vi "Read Data Titles.vi"(8 "error in (no error)":errorcluster, 11 "Device in":refnum<class "Cryo-Con-22C.lvclass">) -> (0 "error out":errorcluster, 2 "Data titles":string[](array[string])=["CRYO CHA"], 3 "Device out":refnum<class "Cryo-Con-22C.lvclass">)   [LabVIEW 2015, in "Cryo-Con-22C.lvclass"]
uses:
  Cryo-Con-22C.lvclass
  Cryo-Con Front Panel Data.ctl
  Cryo-con Heater Ranges.ctl
  Cry-Con Loop Type.ctl
  OO Devices/Device/Read Control Panel Loaded.vi
  OO Devices/Device/Read Controls Snapshot.vi
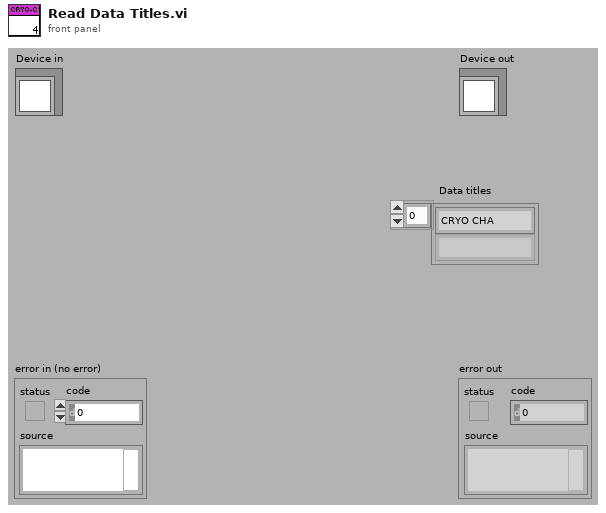
[diagram p1: front panel]
types:
  T1 = typedef "Cryo-Con Front Panel Data.ctl" = cluster{"Channels to measure":string[], "Record heater":bool, "Set point":dbl, "Heater Range":T2, "Control":bool, "Loop type":T3, "Ramp rate,\n K/min":dbl, "Control Channel":string, "P":dbl, "I":dbl, "D":dbl, "Manual %":u16}
  T2 = typedef "Cryo-con Heater Ranges.ctl" = enum16{"25W", "2.5W", "0.25W"}
  T3 = typedef "Cry-Con Loop Type.ctl" = enum16{"Off", "PID", "Manual", "PID Table", "PID Ramp", "PID Table Ramp"}
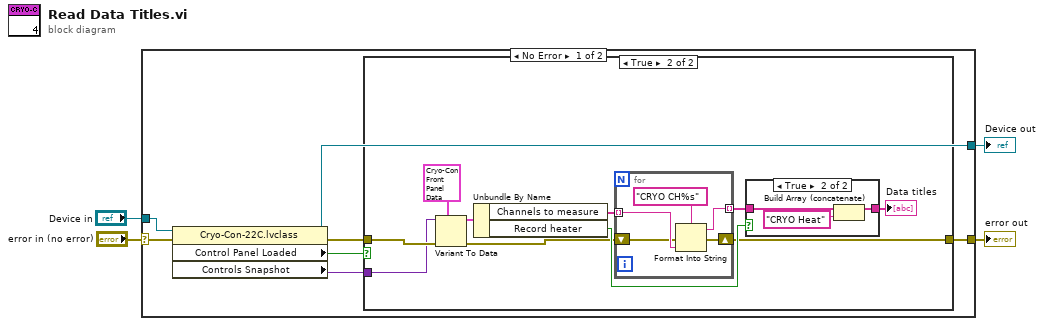
[diagram p0: block diagram]
diagram:
  n1 = case shown="No Error" "error in (no error)" {
    selector: "error in (no error)" -> [w9 w33]
    tunnel: [w7 w33] -> w3
    tunnel: [w10 w32] -> w1
    tunnel: "Device in" -> [w11 w32]
    frame No Error {
      n2 = property class="Cryo-Con-22C.lvclass"(reference=w11, error in=w9) -> (reference out=w10:refnum<class "Cryo-Con-22C.lvclass">, error out=w8:errorcluster, "Control Panel Loaded"=w5:bool, "Controls Snapshot"=w6:variant)
      n3 = case shown="True" w5 {
        tunnel: w8 -> [w12 w21]
        tunnel: [w12 w14] -> w7
        tunnel: w6 -> [_ w13]
        frame False {
        }
        frame True {
          n4 = Variant To Data(error in=w21, type=T1 {"Channels to measure"=["A"], "Record heater"=FALSE, "Set point"=0.0, "Heater Range"=enum."25W", "Control"=FALSE, "Loop type"=enum."Off", "Ramp rate,\n K/min"=1.0, "Control Channel"="A", "P"=0.0, "I"=0.0, "D"=0.0, "Manual %"=0} ("Front Panel Data"), Variant=w13) -> (data=w20:T1, error out=w15:errorcluster)
          n5 = Unbundle By Name(w20) -> ("Channels to measure"=w19:string[], "Record heater"=w18:bool)
          n6 = for {
            tunnel: w19 -> [w30] mode=indexing
            tunnel: [w29] -> w17 mode=indexing
            shift-right: [w27] -> w14
            shift-left: w15 -> [w28]
            n7 = Format Into String(format string="CRYO CH%s", error in=w28, w30) -> (resulting string=w29:string, error out=w27:errorcluster)  [unwired: 1 in]
          }
          n8 = case shown="True" w18 {
            tunnel: w17 -> [w23 w26]
            tunnel: [w23 w25] -> w16
            frame False {
            }
            frame True {
              n9 = Build Array (concatenate)(w26, "CRYO Heat" ("format string")) -> (w25:string[])
            }
          }
          "Data titles" <- w16
        }
      }
    }
    frame Error {
    }
  }
  "error out" <- w3
  "Device out" <- w1
